vi "FPGA_RS232 Read.vi"(0 "Receive":refnum<k21>="Port8/DIOCTL", 1 "FIFO In":refnum<k21>="FIFO_Chan 1", 2 "Mode":bool, 3 "Edge":bool, 5 "data bits (8)":i32=8 min=5 max=8 step=1, 7 "Stop Bit":u16(ring)=10 items=["1.0"=10, "1.5"=15, "2.0"=20], 9 "Invert Polarity?":bool, 11 "Error IN":errorcluster, 12 "Clock Rate":u32=1000, 13 "baud rate":u32=9600, 14 "Clk":refnum<k21>="Port8/DIOCTL") -> (15 "Error OUT":errorcluster)   [LabVIEW 2011]
uses:
  <vilib>/rvi/eio/common/nirviEmuTemplateMethod_errors.vi
  Global_Read.vi
  <vilib>/rvi/DataTransferAndStorage/Container/Common/niFpgaContainerExecOnDevCompGetState.vi
  <vilib>/rvi/FIFO/Fifo_Resource/nirvififoEmulationSetSize.vi
  <vilib>/rvi/DataTransferAndStorage/Container/Common/niFpgaContainerGetUniqueNameForEmu.vi
  <vilib>/rvi/interface/RandomDataEmulation/nirviRandomDataFPGAFIFO.vi
  <vilib>/rvi/interface/RandomDataEmulation/niFpgaRandomDataHandleErrors.vi
  <vilib>/rvi/eio/common/nirviEmuReportErrorAndStop.vi
  <vilib>/eio/EIONode/EIONode.xnode
  <vilib>/rvi/DataTransferAndStorage/Container/XNode/niFpgaContainer.xnode
  <vilib>/rvi/FIFO/Fifo_Resource/niFpgaFifoEmulationRefIn.vi
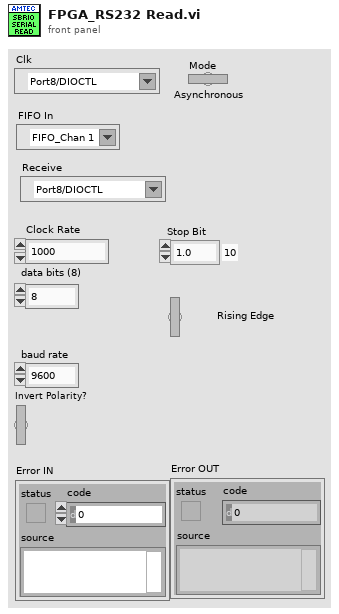
[diagram p1: front panel]
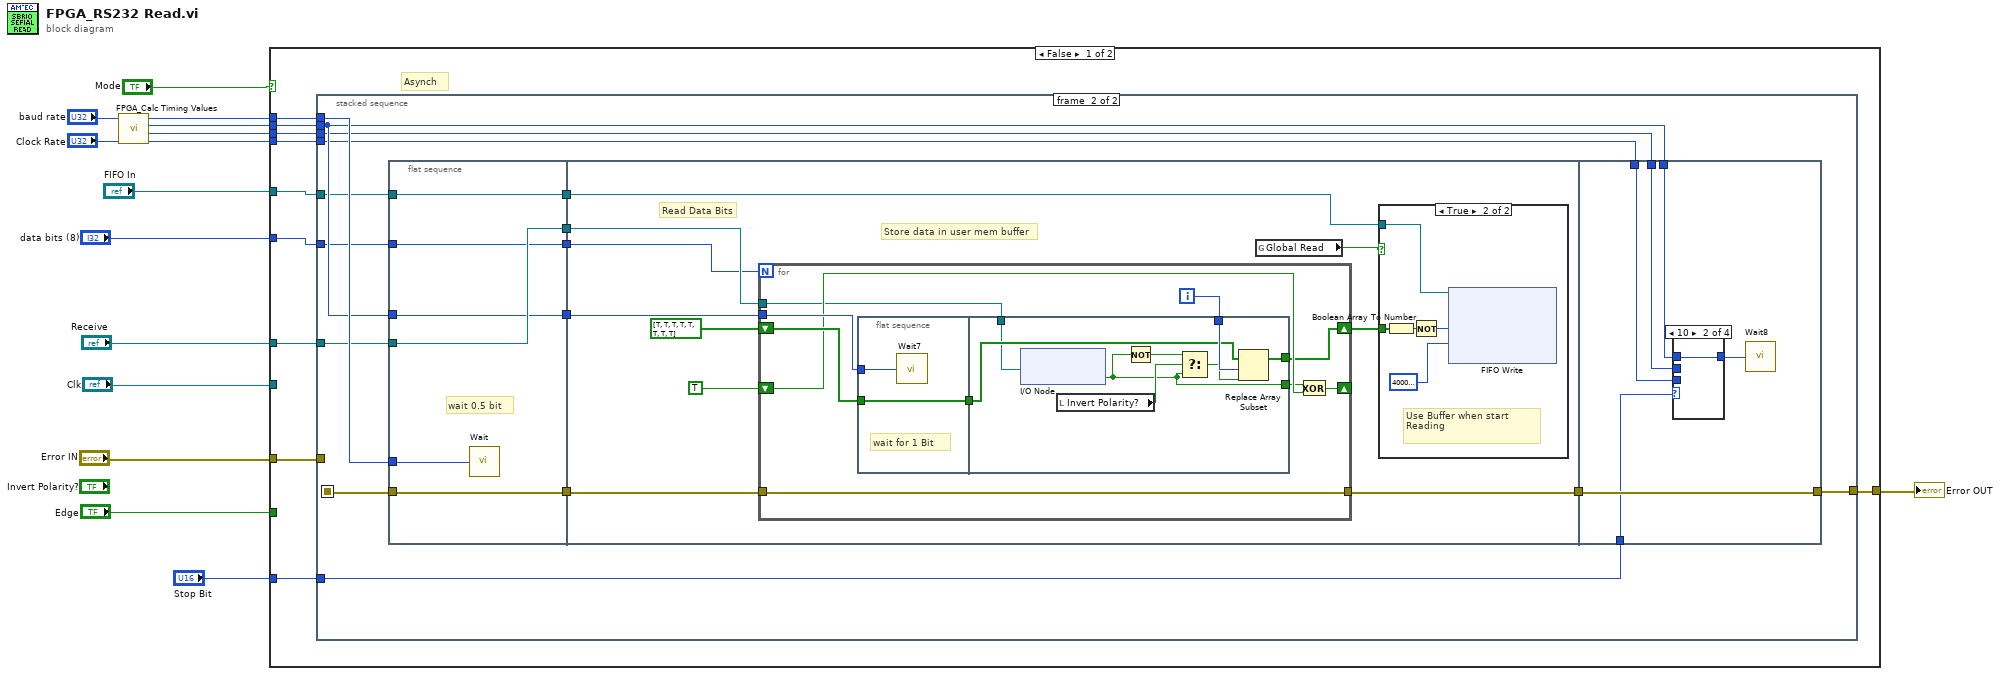
[diagram p0: block diagram]
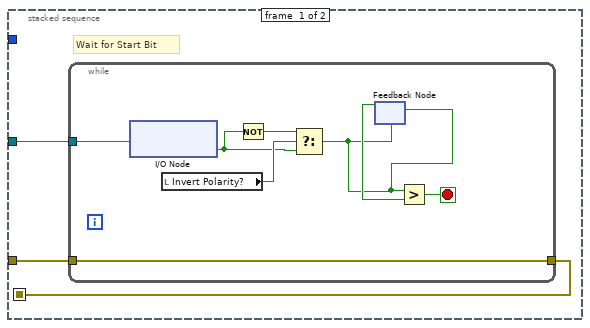
[diagram p2: hidden frame]
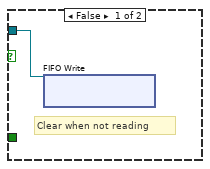
[diagram p3: hidden frame]
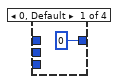
[diagram p4: hidden frame]
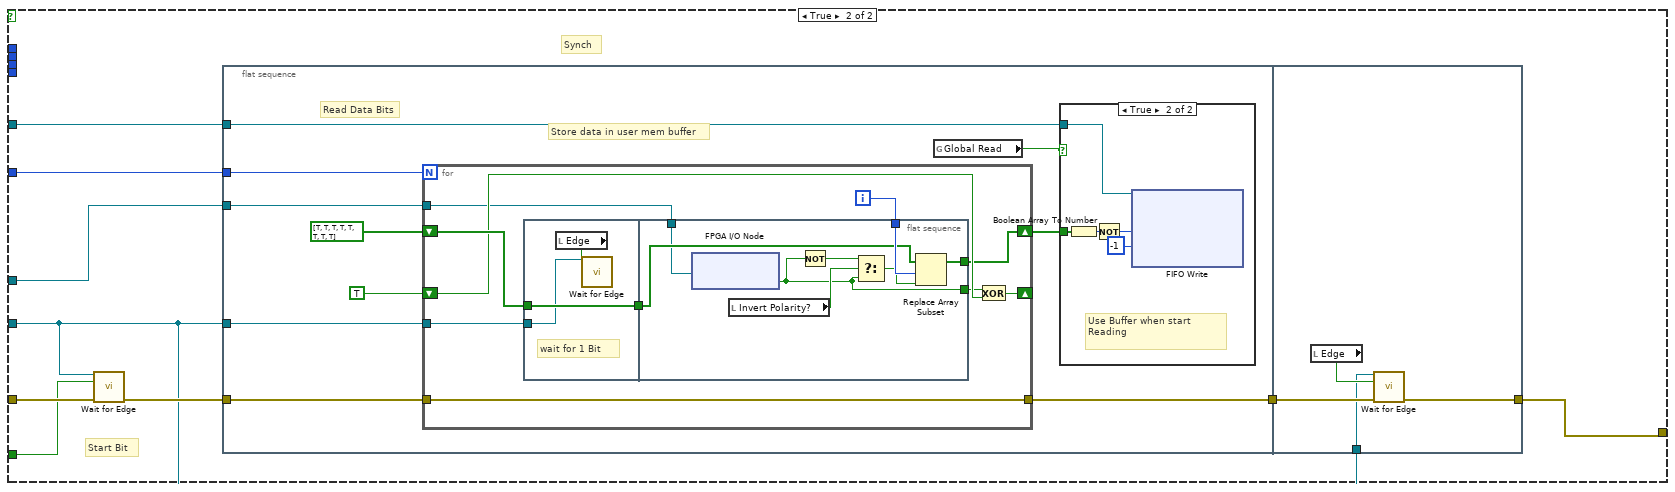
[diagram p7: hidden frame]
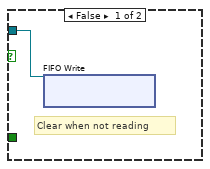
[diagram p8: hidden frame]
diagram:
  n1 = call "FPGA_Calc Timing Values.vi"("FPGA Clock Rate (40000000)"="Clock Rate", "baud rate (1000000)"="baud rate") -> ("Two Bit"=w10:u32, "One and Half Bit"=w11:u32, "One Bit"=w12:u32, "Half Bit"=w13:u32)  [unwired: 2 out]
  n2 = case shown="False" "Mode" {
    tunnel: w13 -> [w25 _]
    tunnel: w12 -> [w24 _]
    tunnel: w11 -> [w23 _]
    tunnel: w10 -> [w22 _]
    tunnel: "Receive" -> [w21 w109]
    tunnel: "Error IN" -> [w20 w113]
    tunnel: [w19 w105] -> w7
    tunnel: "Clk" -> [_ w106]
    tunnel: "Edge" -> [_ w112]
    tunnel: "data bits (8)" -> [w18 w108]
    tunnel: "Stop Bit" -> [w17 _]
    tunnel: "FIFO In" -> [w16 w107]
    frame False {
      # "Asynch"
      n3 = stacked-sequence {
        seq-local: [w26 _] -> [_ w52]
        tunnel: w25 -> [_ w51]
        tunnel: w24 -> [_ w45]
        tunnel: w23 -> [_ w44]
        tunnel: w22 -> [_ w43]
        tunnel: w21 -> [w28 w48]
        tunnel: w20 -> [w27 _]
        tunnel: [_ w42] -> w19
        tunnel: w18 -> [_ w40]
        tunnel: w17 -> [_ w39]
        tunnel: w16 -> [_ w37]
        frame #0 {
          # "Wait for Start Bit"
          n4 = while {
            tunnel: w28 -> [w36]
            tunnel: [w32] -> w26
            tunnel: w27 -> [w32]
            stop <- w30 stop-if-true
            n5 = xnode "I/O Node"("FPGA I/O In"=w36) -> ("I/O Item"=w33:bool)  [unwired: 1 out]
            n6 = local read "Invert Polarity?"() -> (w34:bool)
            n7 = Not(x=w33) -> (.not. x?=w35:bool)
            n8 = Select(t=w35, s=w34, f=w33) -> (s? t:f=w29:bool)
            n9 = feedback-in #1(w29) -> ()
            n10 = feedback #1(w29) -> (w31:bool)
            n11 = Greater?(x=w29, y=w31) -> (0:w30:bool)
          }
        }
        frame #1 {
          n12 = flat-sequence {
            tunnel: w52 -> [w57]
            tunnel: w51 -> [w58]
            tunnel: [w57] -> w50
            tunnel: [w56] -> w49
            tunnel: w48 -> [w56]
            tunnel: [w55] -> w47
            tunnel: w45 -> [w55]
            tunnel: [w54] -> w41
            tunnel: w40 -> [w54]
            tunnel: [w53] -> w38
            tunnel: w37 -> [w53]
            tunnel: w50 -> [w66]
            tunnel: w49 -> [w64]
            tunnel: w47 -> [w62]
            tunnel: [w65] -> w46
            tunnel: w41 -> [w60]
            tunnel: w38 -> [w59]
            tunnel: [w100] -> w42
            tunnel: w46 -> [w100]
            tunnel: w45 -> [w98]
            tunnel: w44 -> [w97]
            tunnel: w43 -> [w96]
            tunnel: w39 -> [w95]
            frame #0 {
              # "wait 0.5 bit"
              n13 = call "Wait"("Count(Ticks)"=w58) -> ()  [unwired: 1 out]
            }
            frame #1 {
              # "Store data in user mem buffer"
              # "Read Data Bits"
              n14 = for {
                N: w60 -> [_]
                shift-right: [w78] -> w67
                shift-left: bool[] [TRUE, TRUE, TRUE, TRUE, TRUE, TRUE, TRUE, TRUE] -> [w84]
                tunnel: w62 -> [w82]
                shift-right: [w81] -> _
                shift-left: TRUE -> [w80]
                tunnel: w64 -> [w76]
                tunnel: w66 -> [w75]
                tunnel: [w75] -> w65
                i -> [w77]
                n15 = flat-sequence {
                  tunnel: w84 -> [w86]
                  tunnel: [w86] -> w83
                  tunnel: w82 -> [w85]
                  tunnel: w77 -> [w94]
                  tunnel: w83 -> [w93]
                  tunnel: [w92] -> w78
                  tunnel: [w87] -> w79
                  tunnel: w76 -> [w91]
                  frame #0 {
                    # "wait for 1 Bit"
                    n16 = call "Wait7"("Count(Ticks)"=w85) -> ()  [unwired: 1 out]
                  }
                  frame #1 {
                    n17 = xnode "I/O Node"("FPGA I/O In"=w91) -> ("I/O Item"=w87:bool)  [unwired: 1 out]
                    n18 = local read "Invert Polarity?"() -> (w90:bool)
                    n19 = Not(x=w87) -> (.not. x?=w89:bool)
                    n20 = Select(t=w89, s=w90, f=w87) -> (s? t:f=w88:bool)
                    n21 = Replace Array Subset(array=w93, new element=w88, index=w94) -> (w92:bool[])
                  }
                }
                n22 = Exclusive Or(1:w80, 2:w79) -> (0:w81:bool)
              }
              n23 = global read "Global_Read.vi" "Global Read"() -> (w61:bool)
              n24 = case shown="True" w61 {
                tunnel: w67 -> [_ w74]
                tunnel: w59 -> [w69 w72]
                frame False {
                  # "Clear when not reading"
                  n25 = xnode ("FIFO Write")("FIFO In"=w69) -> ()  [unwired: 1 out]
                }
                frame True {
                  # "Use Buffer when start \nReading"
                  n26 = Boolean Array To Number(Boolean array=w74) -> (number=w73:u8)
                  n27 = Not(x=w73) -> (.not. x?=w71:u8)
                  n28 = xnode ("FIFO Write")("Element"=w71, "Timeout"=u32 40000000 ("Count(Ticks)"), "FIFO In"=w72) -> ()  [unwired: 2 out]
                }
              }
            }
            frame #2 {
              n29 = case shown="10" w95 {
                tunnel: w98 -> [_ w102 _ _]
                tunnel: w97 -> [_ _ w103 _]
                tunnel: w96 -> [_ _ _ w104]
                tunnel: [u32 0 ("One Bit") w102 w103 w104] -> w99
                frame 0, Default {
                }
                frame 10 {
                }
                frame 15 {
                }
                frame 20 {
                }
              }
              n30 = call "Wait8"("Count(Ticks)"=w99) -> ()  [unwired: 1 out]
            }
          }
        }
      }
    }
    frame True {
      # "Synch"
      # "Start Bit"
      n31 = call "Wait for Edge.vi"("Clk"=w106, "Falling Edge"=w112, "Error IN"=w113) -> ("Error OUT"=w110:errorcluster)  [unwired: 12 in]
      n32 = flat-sequence {
        tunnel: [w120] -> w111
        tunnel: w110 -> [w121]
        tunnel: w109 -> [w119]
        tunnel: w108 -> [w116]
        tunnel: w107 -> [w115]
        tunnel: w106 -> [w114]
        tunnel: [w153] -> w105
        tunnel: w111 -> [w154]
        tunnel: w106 -> [w151]
        frame #0 {
          # "Store data in user mem buffer"
          # "Read Data Bits"
          n33 = for {
            N: w116 -> [_]
            shift-right: [w134] -> w122
            shift-left: bool[] [TRUE, TRUE, TRUE, TRUE, TRUE, TRUE, TRUE, TRUE] -> [w139]
            shift-right: [w137] -> _
            shift-left: TRUE -> [w136]
            tunnel: w119 -> [w132]
            tunnel: w121 -> [w131]
            tunnel: [w131] -> w120
            tunnel: w114 -> [w130]
            i -> [w133]
            n34 = flat-sequence {
              tunnel: w139 -> [w142]
              tunnel: [w142] -> w138
              tunnel: w130 -> [w141]
              tunnel: w133 -> [w150]
              tunnel: w138 -> [w149]
              tunnel: [w148] -> w134
              tunnel: [w143] -> w135
              tunnel: w132 -> [w147]
              frame #0 {
                # "wait for 1 Bit"
                n35 = local read "Edge"() -> (w140:bool)
                n36 = call "Wait for Edge.vi"("Clk"=w141, "Falling Edge"=w140) -> ()  [unwired: 13 in, 1 out]
              }
              frame #1 {
                n37 = xnode "FPGA I/O Node"("FPGA I/O In"=w147) -> ("I/O Item"=w143:bool)  [unwired: 1 out]
                n38 = local read "Invert Polarity?"() -> (w146:bool)
                n39 = Not(x=w143) -> (.not. x?=w145:bool)
                n40 = Select(t=w145, s=w146, f=w143) -> (s? t:f=w144:bool)
                n41 = Replace Array Subset(array=w149, new element=w144, index=w150) -> (w148:bool[])
              }
            }
            n42 = Exclusive Or(1:w136, 2:w135) -> (0:w137:bool)
          }
          n43 = global read "Global_Read.vi" "Global Read"() -> (w117:bool)
          n44 = case shown="True" w117 {
            tunnel: w122 -> [_ w128]
            tunnel: w115 -> [w124 w126]
            frame False {
              # "Clear when not reading"
              n45 = xnode ("FIFO Write")("FIFO In"=w124) -> ()  [unwired: 1 out]
            }
            frame True {
              # "Use Buffer when start \nReading"
              n46 = Boolean Array To Number(Boolean array=w128) -> (number=w127:u8)
              n47 = Not(x=w127) -> (.not. x?=w125:u8)
              n48 = xnode ("FIFO Write")("Element"=w125, "Timeout"=-1, "FIFO In"=w126) -> ()  [unwired: 2 out]
            }
          }
        }
        frame #1 {
          n49 = local read "Edge"() -> (w152:bool)
          n50 = call "Wait for Edge.vi"("Clk"=w151, "Falling Edge"=w152, "Error IN"=w154) -> ("Error OUT"=w153:errorcluster)  [unwired: 12 in]
        }
      }
    }
  }
  "Error OUT" <- w7
